vi "Send status.vi"(8 "error in (no error)":errorcluster, 10 "status":string, 11 "Messenger in":refnum<class "Messenger.lvclass">) -> (0 "error out":errorcluster, 3 "Messenger out":refnum<class "Messenger.lvclass">)   [LabVIEW 2018, in "Messenger.lvclass"]
uses:
  Messenger.lvclass
  Message Queue/Message Cluster.ctl
  Message Queue/Message Queue.lvlib
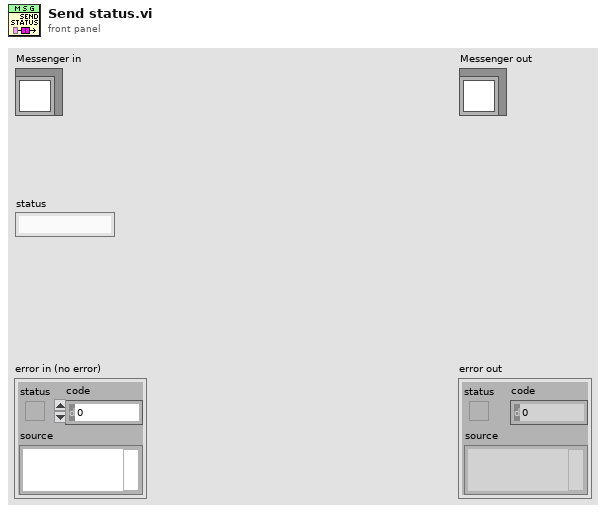
[diagram p1: front panel]
types:
  T1 = typedef "Message Queue.lvlib/Message Cluster.ctl" = cluster{"Message":string, "Message Data":variant}
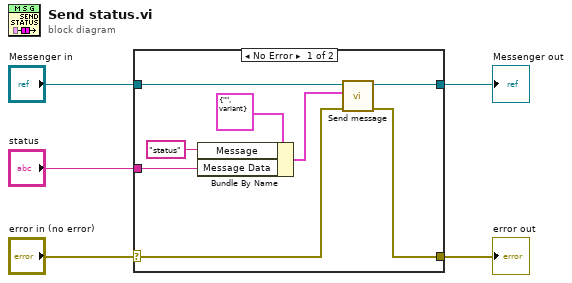
[diagram p0: block diagram]
diagram:
  n1 = case shown="No Error" "error in (no error)" {
    selector: "error in (no error)" -> [w12 w14]
    tunnel: [w6 w14] -> w4
    tunnel: [w11 w15] -> w2
    tunnel: "Messenger in" -> [w13 w15]
    tunnel: "status" -> [w8 _]
    frame No Error {
      n2 = Bundle By Name(cluster=T1 {"Message"="", "Message Data"=variant} ("message"), "Message"="status", "Message Data"=w8) -> (w9:T1)
      n3 = call-dynamic "Send message.vi"("error in (no error)"=w12, "message"=w9, "Messenger in"=w13) -> ("error out"=w6:errorcluster, "Messenger out"=w11:refnum<class "Messenger.lvclass">)  [unwired: 7 in]
    }
    frame Error {
    }
  }
  "error out" <- w4
  "Messenger out" <- w2
